vi "Clear Targets Update.vi"(2 "error in":errorcluster, 3 "Targets Queue":refnum<queue>) -> (0 "error out":errorcluster, 1 "Targets Queue":refnum<queue>)   [LabVIEW 2016]
uses:
  Targets Update.ctl
  Targets Message.ctl
  Targets Info.ctl
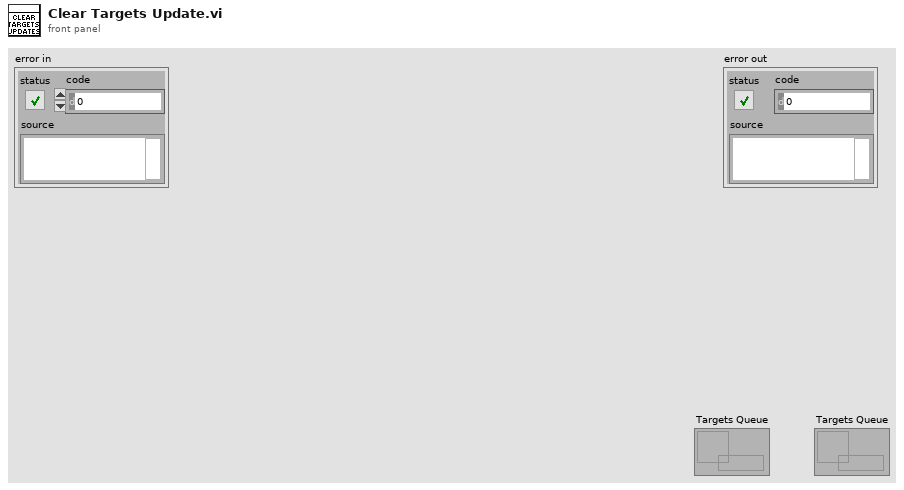
[diagram p1: front panel]
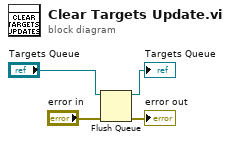
[diagram p0: block diagram]
diagram:
  n1 = Flush Queue(queue="Targets Queue", error in (no error)="error in") -> (queue out=→"Targets Queue":refnum<queue>, error out=→"error out":errorcluster)  [unwired: 1 out]
